vi "Read Channel Timing.vi"(8 "error in":errorcluster, 10 "Data to read in":T1, 11 "Report Viewer in":refnum<class "Report Viewer.lvclass">) -> (0 "error out":errorcluster, 1 "Data to read out":T1, 2 "Channel_Timing":T2, 3 "Report Viewer out":refnum<class "Report Viewer.lvclass">, 4 "Good_Record":bool)   [LabVIEW 2019, in "Report Viewer.lvlib" / "Report Viewer.lvclass"]
uses:
  Library/Report Viewer.lvclass
  Custom Controls/Data to Read.ctl
  Custom Controls/Channel_Timing.ctl
  Library/Report Viewer.lvclass/Report Viewer.ctl
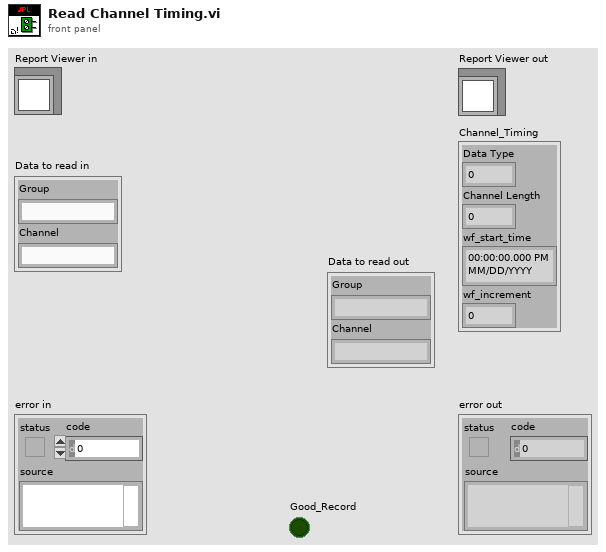
[diagram p1: front panel]
types:
  T1 = typedef "Report Viewer.lvlib/Report Viewer.lvclass/Data to Read.ctl" = cluster{"Group":string, "Channel":string}
  T2 = typedef "Report Viewer.lvlib/Report Viewer.lvclass/Channel_Timing.ctl" = cluster{"Data Type":u16, "Channel Length":u64, "wf_start_time":timestamp, "wf_increment":dbl}
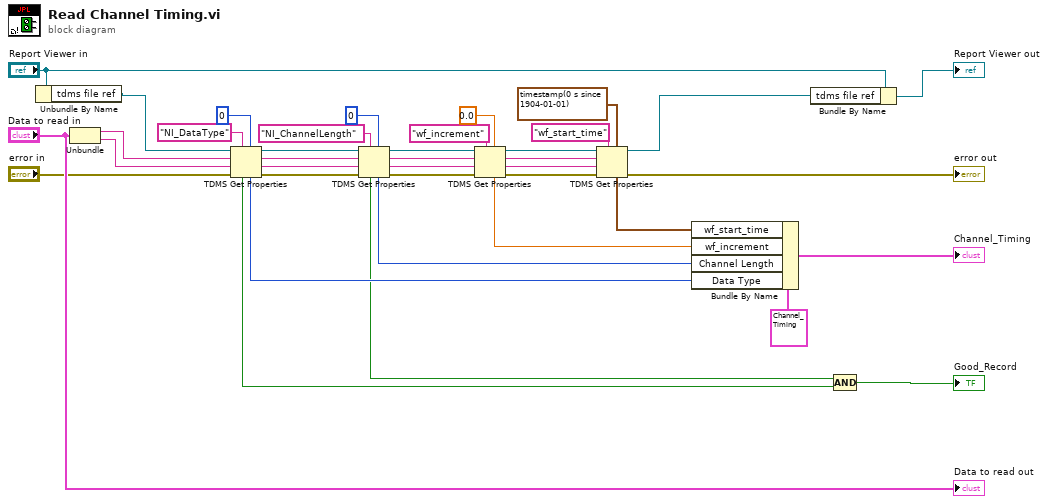
[diagram p0: block diagram]
diagram:
  n1 = Unbundle By Name("Report Viewer in") -> ("tdms file ref"=w4:refnum<k34>)
  n2 = Unbundle("Data to read in") -> ("Group"=w29:string, "Channel"=w28:string)
  n3 = TDMS Get Properties(5:u16 0, 7:"NI_DataType" ("property name"), 8:"error in", 9:w28, 10:w29, 11:w4) -> (0:w33:errorcluster, 1:w36:string, 2:w35:string, 3:w34:refnum<k34>, 4:w19:u16, 6:w6:bool)
  n4 = TDMS Get Properties(5:u64 0, 7:"NI_ChannelLength" ("property name"), 8:w33, 9:w36, 10:w35, 11:w34) -> (0:w26:errorcluster, 1:w23:string, 2:w24:string, 3:w25:refnum<k34>, 4:w18:u64, 6:w7:bool)
  n5 = TDMS Get Properties(5:0.0, 7:"wf_increment" ("property name"), 8:w26, 9:w23, 10:w24, 11:w25) -> (0:w16:errorcluster, 1:w13:string, 2:w14:string, 3:w15:refnum<k34>, 4:w17:dbl)  [unwired: 1 out]
  n6 = TDMS Get Properties(5:timestamp(0 s since 1904-01-01), 7:"wf_start_time" ("property name"), 8:w16, 9:w13, 10:w14, 11:w15) -> (0:→"error out":errorcluster, 3:w2:refnum<k34>, 4:w9:timestamp)  [unwired: 3 out]
  n7 = Bundle By Name(cluster=T2 {"Data Type"=0, "Channel Length"=0, "wf_start_time"=timestamp(0 s since 1904-01-01), "wf_increment"=0.0} ("Data Windowing"), "wf_start_time"=w9, "wf_increment"=w17, "Channel Length"=w18, "Data Type"=w19) -> (→"Channel_Timing":T2)
  n8 = Bundle By Name(cluster="Report Viewer in", "tdms file ref"=w2) -> (→"Report Viewer out":refnum<class "Report Viewer.lvclass">)
  n9 = Compound Arithmetic op=AND(w7, w6) -> (→"Good_Record":bool)
  "Data to read out" <- "Data to read in"
